vi "python_info.vi"() -> ()   [LabVIEW 2024]
uses:
  <vilib>/Python/Open Anaconda Python Session.vi
panel:
  out "module path":path
  out "return value":string
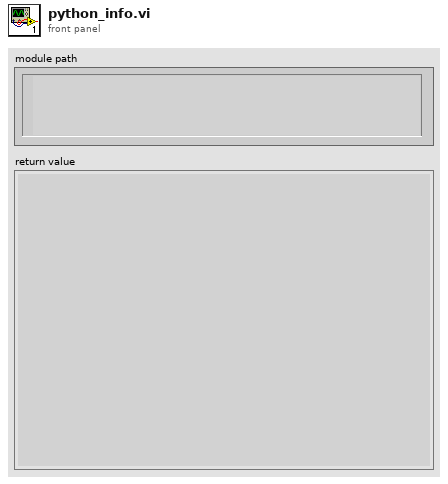
[diagram p1: front panel]
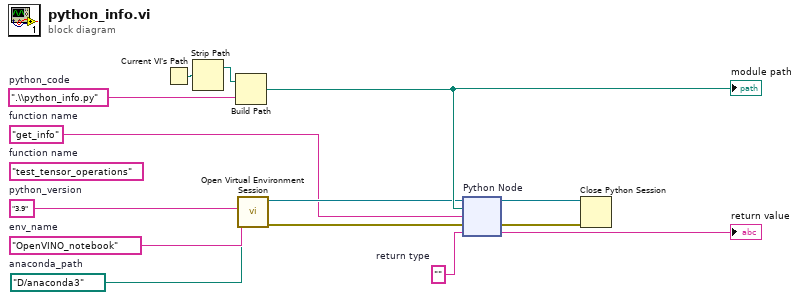
[diagram p0: block diagram]
diagram:
  w4 = path "D:/anaconda3"  # anaconda_path
  w5 = "OpenVINO_notebook"  # env_name
  w9 = ""  # return type
  w6 = "3.9"  # python_version
  (unwired) "test_tensor_operations"  # function name
  w3 = "get_info"  # function name
  w14 = ".\\python_info.py"  # python_code
  n1 = Current VI's Path() -> (path=w2:path)
  n2 = Strip Path(path=w2) -> (stripped path=w1:path)  [unwired: 1 out]
  n3 = Build Path(base path=w1, name or relative path=w14) -> (appended path=w13:path)
  "module path" <- w13
  n4 = call-poly <vilib>:"Open Virtual Environment Session.vi"("Anaconda path"=w4, "Python version"=w6, "Env name"=w5) -> ("error out"=w7:errorcluster, "session out"=w8:refnum<k35>)  [unwired: 7 in]
  n5 = node "Python Node"(w8, w13, w3, w7, w9) -> (w12:refnum<k35>, w11:errorcluster, →"return value":string)  [unwired: 2 out]
  n6 = Close Python Session(session in=w12, error in=w11) -> ()  [unwired: 1 out]
